vi "Create 2d3d Queues.vi"(8 "error in (no error)":errorcluster, 11 "name":string="selectspectrum") -> (0 "error out":errorcluster, 3 "Message Queues":T1)   [LabVIEW 2023, in "Front Panel Message Queue.lvlib"]
doc: "This VI creates and initializes all the message queues for your application. If your application requires more than one message queue, right-click the \"Message Queues\" constant above and select Open Type Def. Add the new Message Queue(s) to the type definition, then initialize them in this VI."
uses:
  Front Panel Message Queue.lvlib
  2d3d Message Queues.ctl
  Message Cluster.ctl
  Enqueue Message (Single).vi
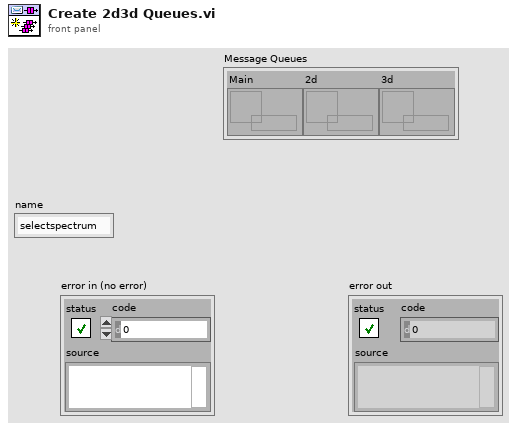
[diagram p1: front panel]
types:
  T1 = typedef "Front Panel Message Queue.lvlib/2d3d Message Queues.ctl" = cluster{"Main":refnum<queue>, "2d":refnum<queue>, "3d":refnum<queue>}
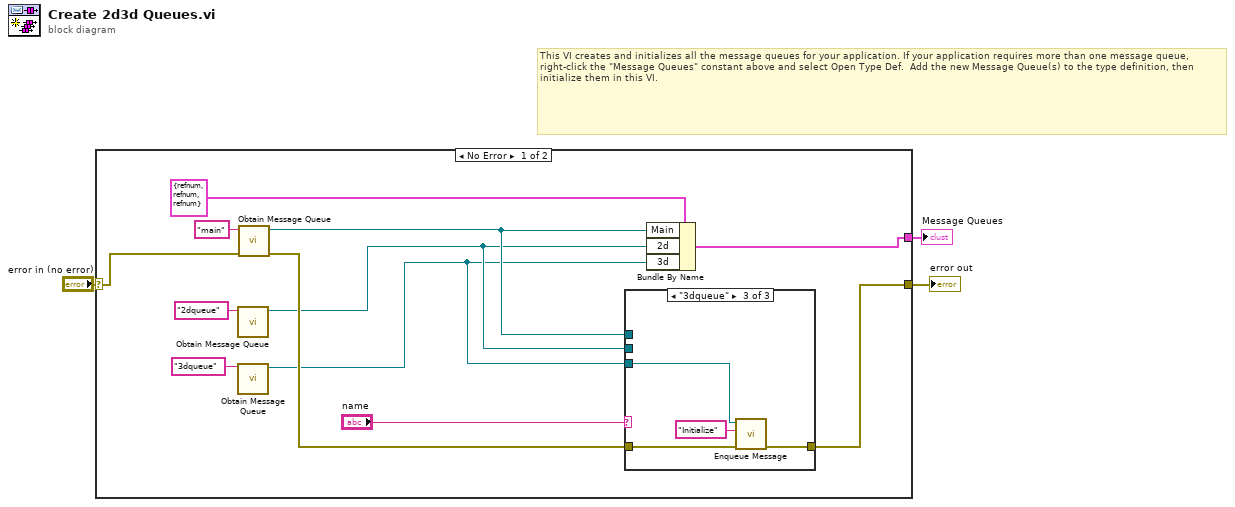
[diagram p0: block diagram]
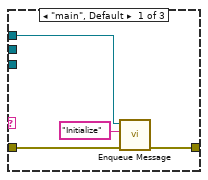
[diagram p2: hidden frame]
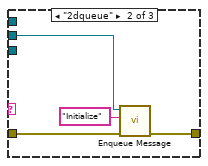
[diagram p3: hidden frame]
diagram:
  # "This VI creates and initializes all the message queues for your application. If your application requires more than one message queue, right-click the \"Message Queues\" constant above and select Open Type Def.  Add the new Message Queue(s) to the type definition, then initialize them in this VI."
  n1 = case shown="No Error" "error in (no error)" {
    selector: "error in (no error)" -> [w12 w28]
    tunnel: [w13 w28] -> w3
    tunnel: [w15 _] -> w1
    frame No Error {
      n2 = call "Obtain Message Queue.vi"("name"="2dqueue") -> ("Message Queue"=w5:refnum<queue>)  [unwired: 9 in, 1 out]
      n3 = call "Obtain Message Queue.vi"("name"="3dqueue") -> ("Message Queue"=w4:refnum<queue>)  [unwired: 9 in, 1 out]
      n4 = call "Obtain Message Queue.vi"("error in (no error)"=w12, "name"="main") -> ("error out"=w14:errorcluster, "Message Queue"=w6:refnum<queue>)  [unwired: 8 in]
      n5 = case shown="\"3dqueue\"" "name" {
        tunnel: w14 -> [w19 w23 w27]
        tunnel: [w18 w22 w26] -> w13
        tunnel: w6 -> [w16 _ _]
        tunnel: w5 -> [_ w20 _]
        tunnel: w4 -> [_ _ w24]
        frame "main", Default {
          n6 = call-poly "Enqueue Message.vi"("error in (no error)"=w19, "Message"="Initialize", "Message Queue"=w16) -> ("error out"=w18:errorcluster)  [unwired: 7 in, 1 out]
        }
        frame "2dqueue" {
          n7 = call-poly "Enqueue Message.vi"("error in (no error)"=w23, "Message"="Initialize", "Message Queue"=w20) -> ("error out"=w22:errorcluster)  [unwired: 7 in, 1 out]
        }
        frame "3dqueue" {
          n8 = call-poly "Enqueue Message.vi"("error in (no error)"=w27, "Message"="Initialize", "Message Queue"=w24) -> ("error out"=w26:errorcluster)  [unwired: 7 in, 1 out]
        }
      }
      n9 = Bundle By Name(cluster=T1 {"Main"=refnum, "2d"=refnum, "3d"=refnum} ("Message Queues"), "Main"=w6, "2d"=w5, "3d"=w4) -> (w15:T1)
    }
    frame Error {
    }
  }
  "error out" <- w3
  "Message Queues" <- w1
